vi "Water on Demand State.vi"(0 "GEA2 Reference In":refnum<k24>, 5 "WOD Expected":T1(ring), 7 "Stand Alone?":bool, 11 "error in":errorcluster) -> (4 "GEA2 Reference Out":refnum<k24>, 6 "WOD Actual":string, 8 "Pass/Fail?":bool, 15 "error out":errorcluster)   [LabVIEW 2016, in "TLMB.lvlib"]
uses:
  Projects/TLMB.lvlib
  Q:/Common/DLLs/GEA3/GeaCommunication.dll
  Common/DLLs/GEA3/GeaCommunication.dll
  Common/LabVIEW GEA2 Toolkit/LabVIEW_GEA2_Toolkit.lvlibp/type defs/Source_Destination.ctl
  Common/LabVIEW GEA2 Toolkit/LabVIEW_GEA2_Toolkit.lvlibp/type defs/ERD Read Data In.ctl
  Common/LabVIEW GEA2 Toolkit/LabVIEW_GEA2_Toolkit.lvlibp/type defs/Data Type.ctl
  Common/LabVIEW GEA2 Toolkit/LabVIEW_GEA2_Toolkit.lvlibp
panel:
  in  "GEA Inputs":T2={"Source"=228, "Destination"=35} {"Destination" format="%.0x"; "Source" format="%.0x"}
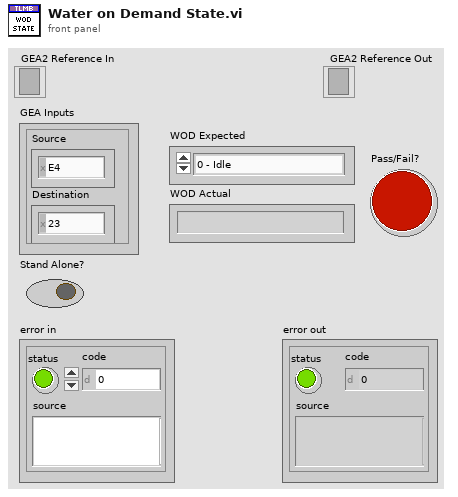
[diagram p1: front panel]
types:
  T1 = enum16{"0 - Idle", "1 - Fill Active", "2 - Fill Pending", "3 - Fill Paused", "4 - Fill Soak", "5 - Full", "6 - Disarmed Selected", "7 - Disarmed Deselected", "8 - Draining"}
  T2 = typedef "LabVIEW_GEA2_Toolkit.lvlibp/Source_Destination.ctl" = cluster{"Source":u8, "Destination":u8}
  T3 = typedef "LabVIEW_GEA2_Toolkit.lvlibp/ERD Read Data In.ctl" = cluster{"ERD Number":u16, "Data Type":T4}
  T4 = typedef "LabVIEW_GEA2_Toolkit.lvlibp/Data Type.ctl" = enum16{"string", "boolean", "uint8_t", "uint16_t", "uint32_t", "uint64_t", "int8_t", "int16_t", "int32_t", "int64_t"}
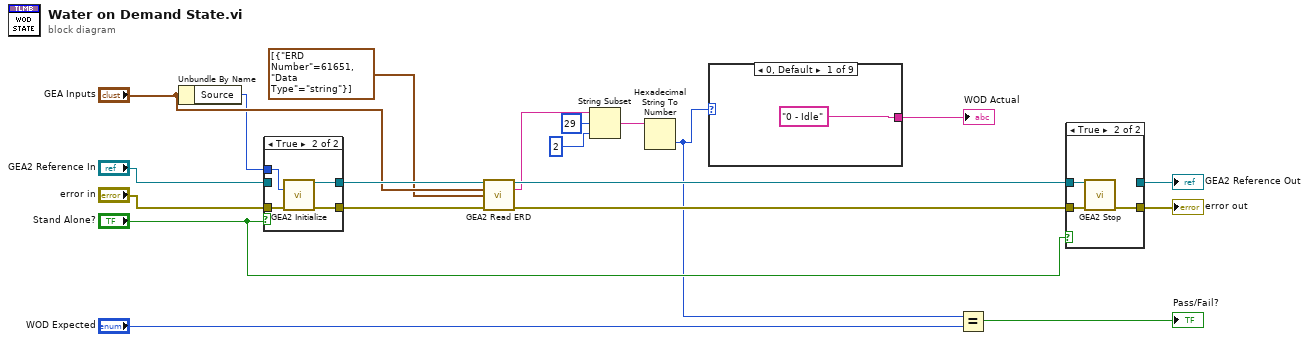
[diagram p0: block diagram]
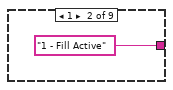
[diagram p2: hidden frame]
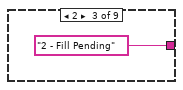
[diagram p3: hidden frame]
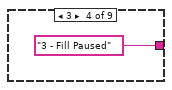
[diagram p4: hidden frame]
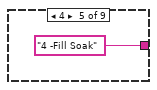
[diagram p5: hidden frame]
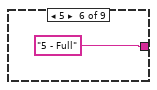
[diagram p6: hidden frame]
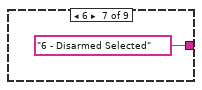
[diagram p7: hidden frame]
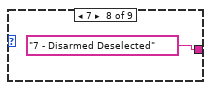
[diagram p8: hidden frame]
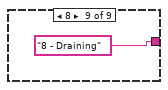
[diagram p9: hidden frame]
diagram:
  n1 = Unbundle By Name("GEA Inputs") -> ("Source"=w12:u8)
  n2 = case shown="True" "Stand Alone?" {
    tunnel: "GEA2 Reference In" -> [w22 _]
    tunnel: [w22 w26] -> w20
    tunnel: "error in" -> [w21 w25]
    tunnel: [w21 w24] -> w18
    tunnel: w12 -> [_ w23]
    frame False {
    }
    frame True {
      n3 = call "GEA2 Initialize.vi"("Source Address"=w23, "error in"=w25) -> ("GEA2 Reference Out"=w26:refnum<k24>, "error out"=w24:errorcluster)  [unwired: 11 in, 1 out]
    }
  }
  n4 = call "GEA2 Read ERD.vi"("GEA2 Reference In"=w20, "GEA Inputs"="GEA Inputs", "Read ERD List"=T3[] [{"ERD Number"=61651, "Data Type"=enum."string"}], "Error In"=w18) -> ("GEA2 Reference Out"=w15:refnum<k24>, "Raw Data Out"=w8:string, "Error Out"=w17:errorcluster)  [unwired: 8 in, 1 out]
  n5 = String Subset(string=w8, offset (0)=29, length (rest)=2 ("length (rest)")) -> (substring=w5:string)
  n6 = Hexadecimal String To Number(string=w5) -> (number=w2:u32)  [unwired: 2 in, 1 out]
  n7 = case shown="0, Default" w2 {
    tunnel: ["0 - Idle" "1 - Fill Active" "2 - Fill Pending" "3 - Fill Paused" "4 -Fill Soak" "5 - Full" "6 - Disarmed Selected" "7 - Disarmed Deselected" "8 - Draining"] -> w3
    frame 0, Default {
    }
    frame 1 {
    }
    frame 2 {
    }
    frame 3 {
    }
    frame 4 {
    }
    frame 5 {
    }
    frame 6 {
    }
    frame 7 {
    }
    frame 8 {
    }
  }
  "WOD Actual" <- w3
  n8 = Equal?(x=w2, y="WOD Expected") -> (x = y?=→"Pass/Fail?":bool)
  n9 = case shown="True" "Stand Alone?" {
    tunnel: w17 -> [w37 w40]
    tunnel: [w37 w39] -> w16
    tunnel: w15 -> [w36 w38]
    tunnel: [w36 _] -> w14
    frame False {
    }
    frame True {
      n10 = call "GEA2 Stop.vi"("GEA2 Reference In"=w38, "Error In"=w40) -> ("Error Out"=w39:errorcluster)  [unwired: 13 in]
    }
  }
  "error out" <- w16
  "GEA2 Reference Out" <- w14
